vi "Send Set Polling Message Msg.vi"(8 "error in (no error)":errorcluster, 10 "Polling Message":refnum<class "~Message.lvclass">, 11 "Message Queue in":refnum<queue>) -> (0 "error out":errorcluster, 3 "Message Queue out":refnum<queue>)   [LabVIEW 2024, in "Zero Timeout Message Handler.lvlib" / "Set Polling Message Msg.lvclass"]
uses:
  Set Polling Message Msg.lvclass
  ~Message/~Message.lvclass
  Set Polling Message Msg.lvclass/Set Polling Message Msg.ctl
  C:/Users/uspoaotto/OneDrive - Oregon Tool/Desktop/working copies/zeroTimeoutMessageHandler/src/Zero Timeout Message Handler/Set Timeout Message Msg/Set Polling Message Msg.lvclass
  C:/Users/uspoaotto/OneDrive - Oregon Tool/Desktop/working copies/zeroTimeoutMessageHandler/src/Zero Timeout Message Handler/~Message/~Message.lvclass
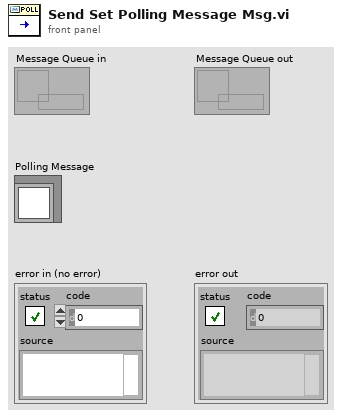
[diagram p1: front panel]
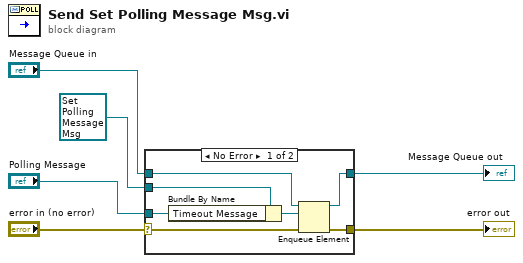
[diagram p0: block diagram]
diagram:
  n1 = case shown="No Error" "error in (no error)" {
    selector: "error in (no error)" -> [w12 w15]
    tunnel: [w11 w15] -> w5
    tunnel: "Message Queue in" -> [w13 w14]
    tunnel: [w10 w14] -> w3
    tunnel: refnum<class "Set Polling Message Msg.lvclass"> refnum ("Zero Timeout Message Handler.lvlib:Set Timeout Message Msg.lvclass") -> [w9 _]
    tunnel: "Polling Message" -> [w8 _]
    frame No Error {
      n2 = Bundle By Name(cluster=w9, "Timeout Message"=w8) -> (w7:refnum<class "Set Polling Message Msg.lvclass">)
      n3 = Enqueue Element(queue=w13, element=w7, error in (no error)=w12) -> (queue out=w10:refnum<queue>, error out=w11:errorcluster)  [unwired: 1 in, 1 out]
    }
    frame Error {
    }
  }
  "error out" <- w5
  "Message Queue out" <- w3
